vi "qp_initial working set from history.vi"(0 "previous working set indices":i32[](array[numeric]), 5 "inequalities":T1, 7 "inequality constants":dbl[](array[numeric]), 11 "A":dbl[][](array[numeric]), 13 "b":dbl[](array[numeric])) -> (4 "current working set indices":i32[](array[numeric]), 6 "A working set":T1, 8 "b working set":dbl[](array[numeric]), 10 "not working set indices out":i32[](array[numeric]), 14 "b not working set":dbl[](array[numeric]), 15 "A not working set":T1)   [LabVIEW 2010, in "NI_Gmath.lvlib"]
uses:
  NI_Gmath.lvlib
  RealMatrix.ctl
  Ramp Pattern by Samples.vi
  Real Matrix Rank.vi
  NI_AALPro.lvlib
  NI_AALBase.lvlib
  NI_Matrix.lvlib
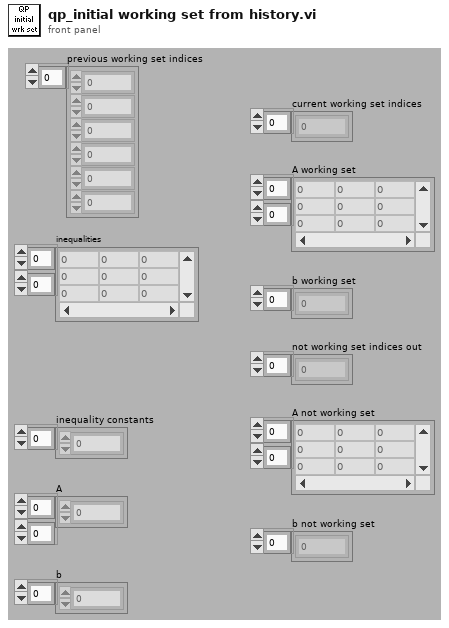
[diagram p1: front panel]
types:
  T1 = typedef "NI_Matrix.lvlib/RealMatrix.ctl" = dbl[][]
  T2 = enum32{"move out of working set", "move into working set", "unchanged working set"}
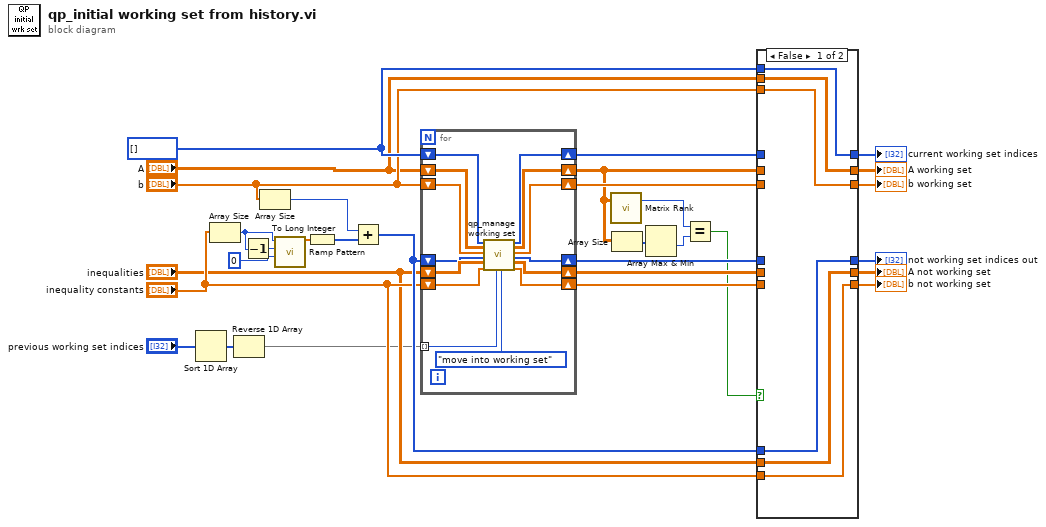
[diagram p0: block diagram]
diagram:
  w14 = i32[] [] ("working set indices out")
  n1 = Sort 1D Array(array="previous working set indices") -> (sorted array=w8:i32[])
  n2 = Array Size(array="inequality constants") -> (size(s)=w17:i32)
  n3 = Reverse 1D Array(array=w8) -> (reversed array=w6:i32[])
  n4 = Decrement(x=w17) -> (x-1=w19:i32)
  n5 = Array Size(array="b") -> (size(s)=w15:i32)
  n6 = call-poly "Ramp Pattern.vi"("start"=0, "end"=w19, "samples"=w17) -> ("Ramp Pattern"=w18:dbl[])  [unwired: 7 in, 1 out]
  n7 = To Long Integer(number=w18) -> (32bit integer=w16:i32[])
  n8 = Add(x=w15, y=w16) -> (x+y=w12:i32[])
  n9 = for {
    tunnel: w6 -> [w45] mode=indexing
    shift-right: [w40] -> w5
    shift-left: "A" -> [w44]
    shift-right: [w39] -> w22
    shift-left: "b" -> [w43]
    shift-right: [w38] -> w24
    shift-left: "inequalities" -> [w42]
    shift-right: [w37] -> w25
    shift-left: "inequality constants" -> [w41]
    shift-right: [w33] -> w21
    shift-left: w14 -> [w34]
    shift-right: [w32] -> w23
    shift-left: w12 -> [w35]
    n10 = call "qp_manage working set.vi"("working set indices in"=w34, "A working set"=w44, "b working set"=w43, "not working set indices in"=w35, "A not working set"=w42, "b not working set"=w41, "index"=w45, "direction"=T2."move into working set") -> ("working set indices out"=w33:i32[], "A working set"=w40:T1, "b working set"=w39:dbl[], "not working set indices out"=w32:i32[], "A not working set"=w38:T1, "b not working set"=w37:dbl[])  [unwired: 6 in]
  }
  n11 = call-poly "Matrix Rank.vi"("Input Matrix"=w5) -> ("rank"=w3:i32)  [unwired: 1 in, 1 out]
  n12 = Array Size(array=w5) -> (size(s)=w4:i32[])
  n13 = Array Max & Min(array=w4) -> (min value=w2:i32)  [unwired: 3 out]
  n14 = Equal?(x=w3, y=w2) -> (x = y?=w1:bool)
  n15 = case shown="False" w1 {
    tunnel: w21 -> [_ w57]
    tunnel: w5 -> [_ w56]
    tunnel: w22 -> [_ w55]
    tunnel: w23 -> [_ w54]
    tunnel: w24 -> [_ w53]
    tunnel: w25 -> [_ w52]
    tunnel: [w51 w57] -> w26
    tunnel: [w50 w56] -> w27
    tunnel: [w49 w55] -> w28
    tunnel: [w48 w54] -> w29
    tunnel: [w47 w53] -> w30
    tunnel: [w46 w52] -> w31
    tunnel: w14 -> [w51 _]
    tunnel: "A" -> [w50 _]
    tunnel: "b" -> [w49 _]
    tunnel: w12 -> [w48 _]
    tunnel: "inequalities" -> [w47 _]
    tunnel: "inequality constants" -> [w46 _]
    frame False {
    }
    frame True {
    }
  }
  "b not working set" <- w31
  "A not working set" <- w30
  "not working set indices out" <- w29
  "b working set" <- w28
  "A working set" <- w27
  "current working set indices" <- w26
